vi "Unix ns to Double.vi"(3 "unix ns":i64) -> (1 "Timestamp":dbl format="%<%H:%M:%S%3u\n%m/%d>T")   [LabVIEW 2020, in "Vecto.lvlib"]
uses:
  Vecto.lvlib
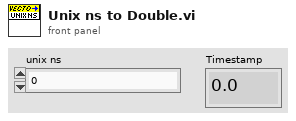
[diagram p1: front panel]
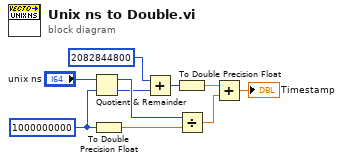
[diagram p0: block diagram]
diagram:
  w9 = i64 1000000000 ("y")
  n1 = Quotient & Remainder(x="unix ns", y=w9) -> (x-y*floor(x/y)=w7:i64, floor(x/y)=w2:i64)
  n2 = To Double Precision Float(number=w9) -> (double precision float=w8:dbl)
  n3 = Add(x=i64 2082844800 ("y"), y=w2) -> (x+y=w1:i64)
  n4 = To Double Precision Float(number=w1) -> (double precision float=w6:dbl)
  n5 = Divide(x=w7, y=w8) -> (x/y=w5:dbl)
  n6 = Add(x=w6, y=w5) -> (x+y=→"Timestamp":dbl)
